vi "Main.vi"() -> ()   [LabVIEW 2020, in "ChromTech Next Gen Pump.lvlib"]
uses:
  ChromTech Next Gen Pump.lvlib
  process loops/Instrument Manager/Instrument State.ctl
  process loops/UI Manager/Data Display Loop Data.ctl
  process loops/Logging/Logging Configuration.ctl
  process loops/UI Manager/UI Data.ctl
  process loops/UI Manager/UI Display State.ctl
  Typedefs/System Control Data.ctl
  <vilib>/Utility/error.llb/Error Cluster From Error Code.vi
  <vilib>/ErrorRing/Error Ring.xnode
  support/Message Queue/Message Queue.lvlib
  support/User Event - Stop/User Event - Stop.lvlib
  process loops/Instrument Manager/Instrument Manager.lvlib
  process loops/Acquisition/Acquisition.lvlib
  process loops/Remote Connection Manager/Remote Connection Manager.lvlib
  process loops/Logging/Logging.lvlib
panel:
  in  "Time Interval (sec)":i32=1200
  out "Data Graph":cluster{timestamp[], dbl[]}[](graph)
  in  "Config Log Btn":bool
  in  "Sampling rate\n(sec/sample)":dbl=5.0 min=0.1 step=0.1
  in  "Log Data":bool
  in  "Stop Btn":bool=TRUE
  in  "Run Btn":bool
  out "Data Ind":dbl format="%d psi"
  in  "Flow Rate (mL/min)":dbl format="%.3f"
  out "VISA resource":refnum<visa-resource-name>
  # "Pump Control Panel"
  # "Config"
  # "Pump Control"
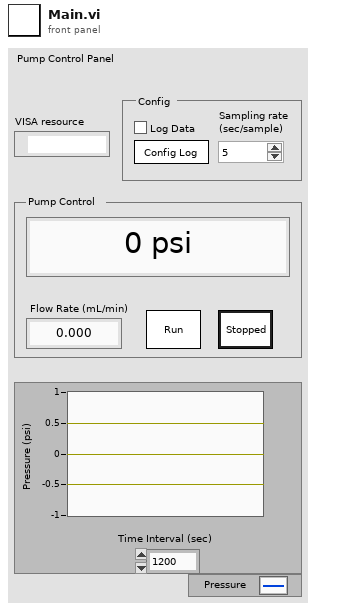
[diagram p1: front panel]
types:
  T1 = typedef "ChromTech Next Gen Pump.lvlib/Data Display Loop Data.ctl" = cluster{"Data Timestamps":timestamp[], "Data Values":dbl[], "Previous Run State":bool}
  T2 = typedef "ChromTech Next Gen Pump.lvlib/Instrument Manager.lvlib/Instrument State.ctl" = cluster{"VISA Resource":refnum<visa-resource-name>, "Flow Rate":dbl, "Running":bool, "Running Since":timestamp, "Pressure Data Point":cluster{"Time Stamp":timestamp, "Value":dbl}, "Upper Pressure Fault":bool, "Lower Pressure Fault":bool, "Motor Stall Fault":bool, "Sampling Rate (sec/sample)":dbl, "Retry Attempts":i32, "Fast Comms":bool}
  T3 = typedef "ChromTech Next Gen Pump.lvlib/Message Queue.lvlib/All Message Queues.ctl" = cluster{"System Control":refnum<queue>, "Instrument":refnum<queue>, "Remote":refnum<queue>, "UI":refnum<queue>, "Acquisition":refnum<queue>, "Logging":refnum<queue>}
  T4 = typedef "ChromTech Next Gen Pump.lvlib/UI Display State.ctl" = enum16{"Shown", "Hidden"}
  T5 = enum8{"Enabled", "Disabled", "Disabled and Grayed Out"}
  T6 = typedef "ChromTech Next Gen Pump.lvlib/UI Data.ctl" = cluster{"VISA Resource Ind":refnum<vi>, "Setpoint Ctl":refnum<vi>, "Run Btn":refnum<vi>, "Stop Btn":refnum<vi>, "Data Ind":refnum<vi>, "Log Data":refnum<vi>, "Config Log Btn":refnum<vi>, "Sampling rate\n(sec/sample)":refnum<vi>, "Data Graph":refnum<vi>}
  T7 = typedef "ChromTech Next Gen Pump.lvlib/Logging.lvlib/Logging Configuration.ctl" = cluster{"Log Directory Path":path, "Log File Path":path, "Log File Prefix":string, "Log File Extension":string, "File Delimiter":string, "Header Info":string[][], "Channels":string[], "Log Instrument Runs":bool}
  T8 = typedef "ChromTech Next Gen Pump.lvlib/System Control Data.ctl" = cluster{"Example Value <Replace Me>":dbl, "Log Runs":bool, "Clone":bool}
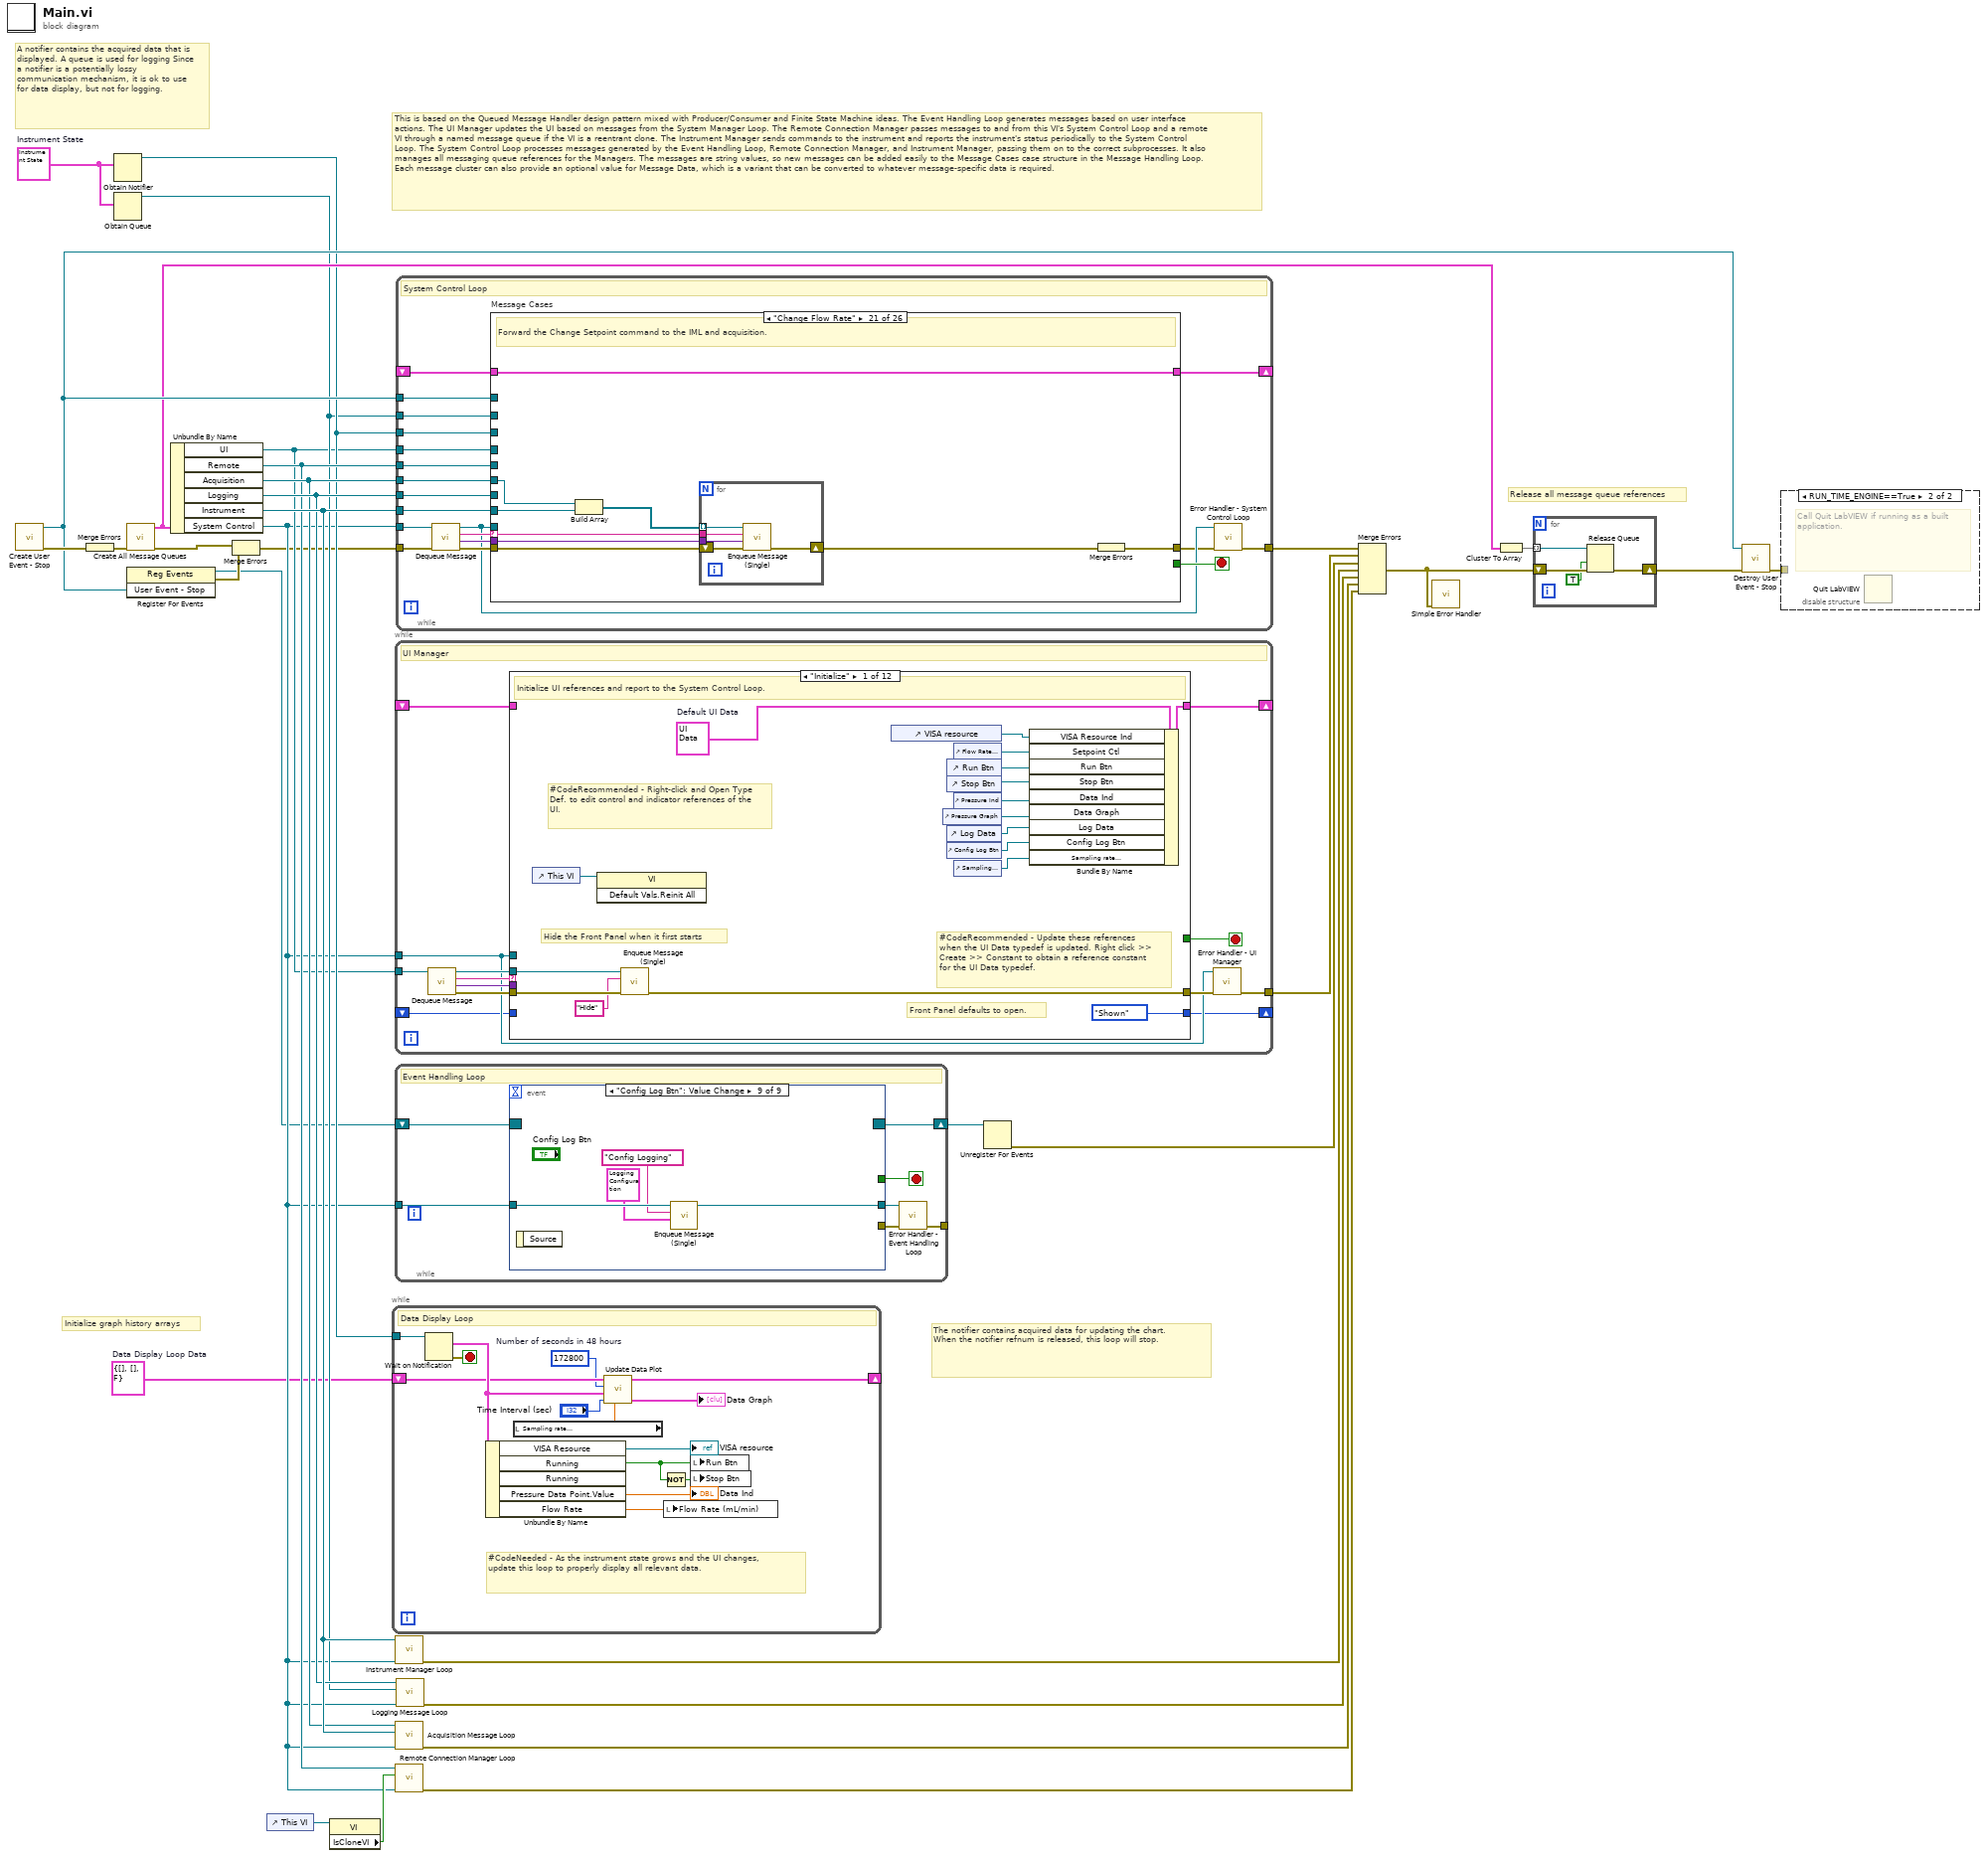
[diagram p0: block diagram]
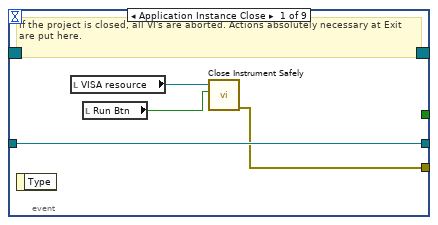
[diagram p2: hidden frame]
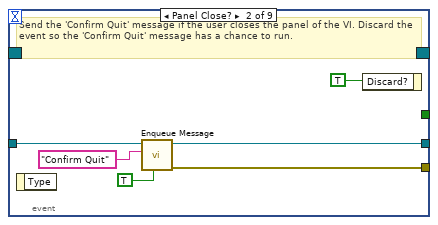
[diagram p3: hidden frame]
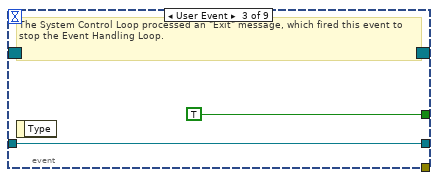
[diagram p4: hidden frame]
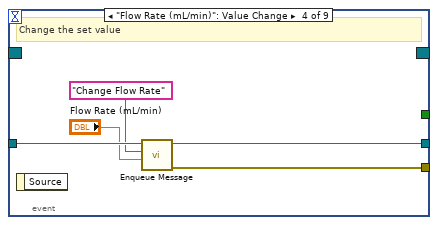
[diagram p5: hidden frame]
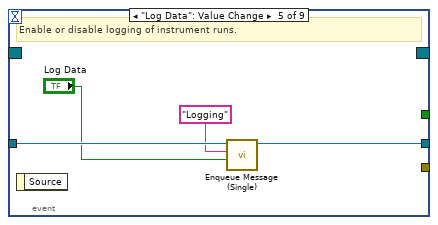
[diagram p6: hidden frame]
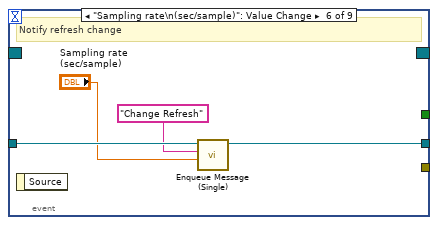
[diagram p7: hidden frame]
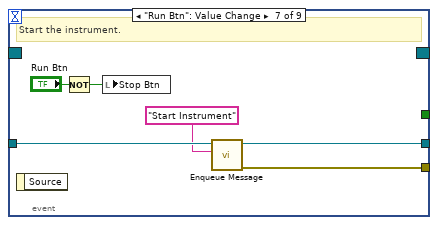
[diagram p8: hidden frame]
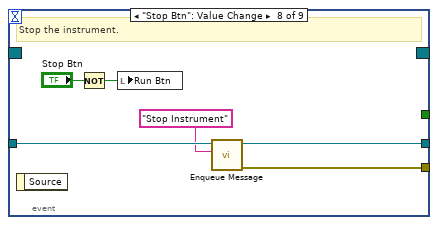
[diagram p9: hidden frame]
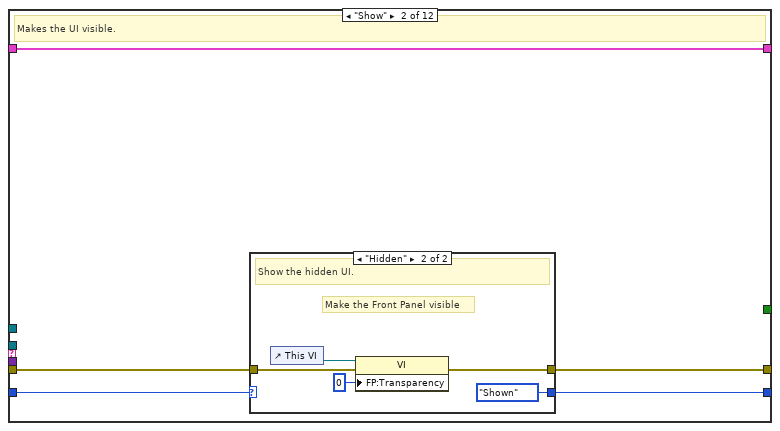
[diagram p10: hidden frame]
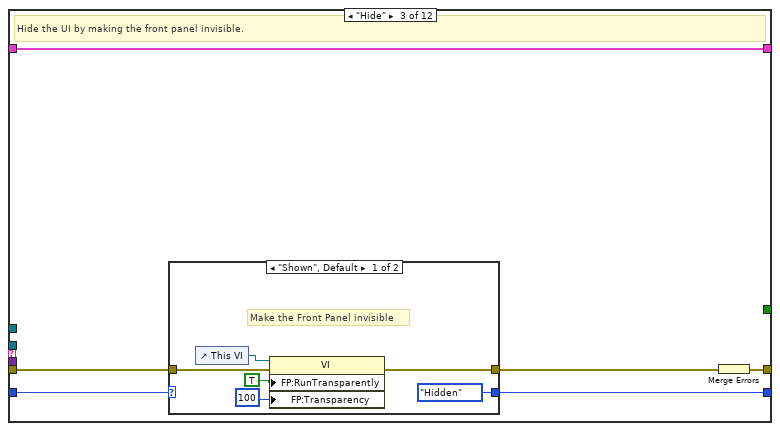
[diagram p12: hidden frame]
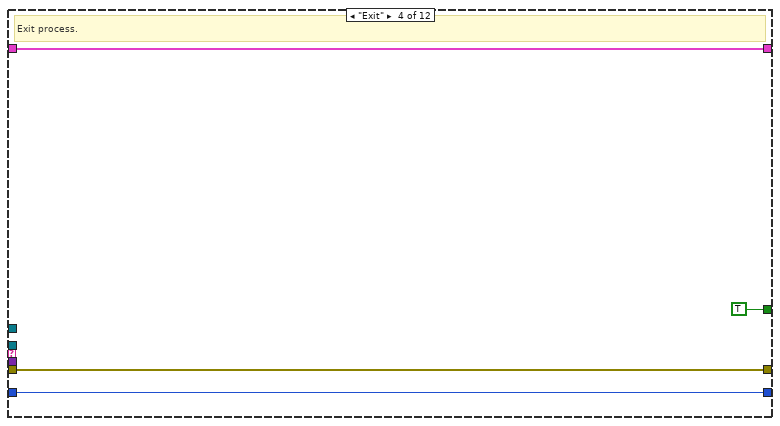
[diagram p14: hidden frame]
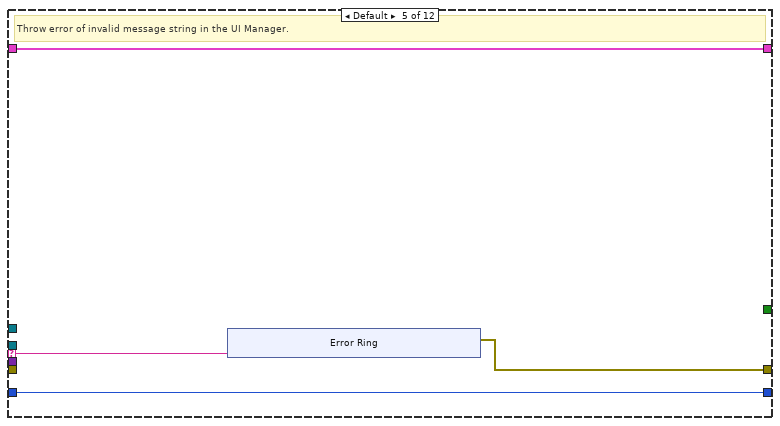
[diagram p15: hidden frame]
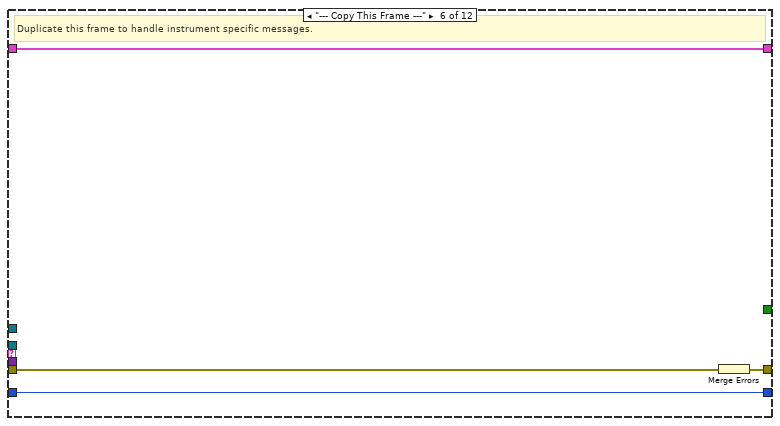
[diagram p16: hidden frame]
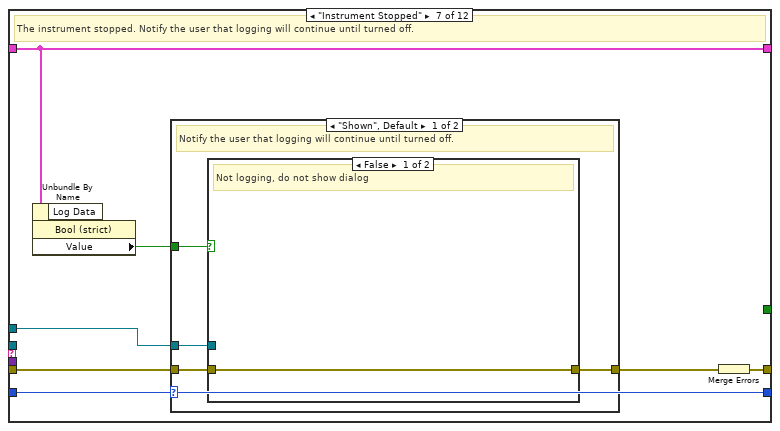
[diagram p17: hidden frame]
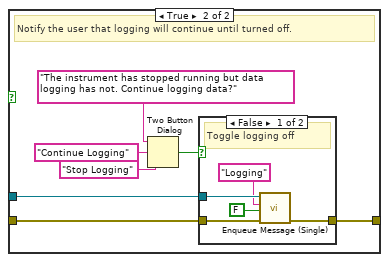
[diagram p18: hidden frame]
diagram:
  w1 = T1 {"Data Timestamps"=[], "Data Values"=[], "Previous Run State"=FALSE}  # Data Display Loop Data
  w7 = T2 {"VISA Resource"="", "Flow Rate"=0.0, "Running"=FALSE, "Running Since"=timestamp(0 s since 1904-01-01), "Pressure Data Point"={"Time Stamp"=timestamp(0 s since 1904-01-01), "Value"=0.0}, "Upper Pressure Fault"=FALSE, "Lower Pressure Fault"=FALSE, "Motor Stall Fault"=FALSE, "Sampling Rate (sec/sample)"=0.0, "Retry Attempts"=0, "Fast Comms"=FALSE}  # Instrument State
  # "Initialize graph history arrays"
  # "A notifier contains the acquired data that is displayed. A queue is used for logging Since a notifier is a potentially lossy communication mechanism, it is ok to use for data display, but not for logging."
  # "The notifier contains acquired data for updating the chart. When the notifier refnum is released, this loop will stop."
  # "Release all message queue references"
  # "This is based on the Queued Message Handler design pattern mixed with Producer/Consumer and Finite State Machine ideas. The Event Handling Loop generates messages based on user interface actions. The UI Manager updates the UI based on messages from the System Manager Loop. The Remote Connection Manager passes messages to and from this VI's System Control Loop and a remote VI through a named message queue if the VI is a reentrant clone. The Instrument Manager sends commands to the instrument and reports the instrument's status periodically to the System Control Loop. The System Control Loop processes messages generated by the Event Handling Loop, Remote Connection Manager, and Instrument Manager, passing them on to the correct subprocesses. It also manages all messaging queue references for the Managers. The messages are string values, so new messages can be added easily to the Message Cases case structure in the Message Handling Loop.  Each message cluster can also provide an optional value for Message Data, which is a variant that can be converted to whatever message-specific data is required."
  n1 = call "Create User Event - Stop.vi"() -> ("error out"=w26:errorcluster, "User Event - Stop"=w22:refnum<user-event>)  [unwired: 10 in]
  n2 = Merge Errors(w26) -> (w25:errorcluster)
  n3 = Obtain Notifier(notification data type=w7) -> (notifier out=w8:refnum<notifier>)  [unwired: 3 in, 2 out]
  n4 = Obtain Queue(element data type=w7) -> (queue out=w6:refnum<queue>)  [unwired: 4 in, 2 out]
  n5 = call "Create All Message Queues.vi"("error in (no error)"=w25) -> ("error out"=w28:errorcluster, "Message Queues out"=w11:T3)  [unwired: 9 in]
  n6 = register-events(w22) -> (reference out=w2:refnum<event-registration>, error out=w13:errorcluster)  [unwired: 2 in]
  n7 = Unbundle By Name(w11) -> ("UI"=w5:refnum<queue>, "Remote"=w29:refnum<queue>, "Acquisition"=w30:refnum<queue>, "Logging"=w31:refnum<queue>, "Instrument"=w32:refnum<queue>, "System Control"=w4:refnum<queue>)
  n8 = Merge Errors(w28, w13) -> (w3:errorcluster)
  n9 = control-ref of="This VI"() -> (w21:refnum<vi>)
  n10 = property class="VI"(reference=w21) -> ("IsCloneVI"=w20:bool)  [unwired: 1 in, 2 out]
  n11 = while "Data Display Loop" {
    tunnel: w8 -> [w46]
    shift-right: [w36] -> _
    shift-left: w1 -> [w37]
    stop <- w45 stop-if-true
    w33 = 172800  # Number of seconds in 48 hours
    # "#CodeNeeded - As the instrument state grows and the UI changes, update this loop to properly display all relevant data."
    # "Data Display Loop"
    n12 = Wait on Notification(notifier=w46) -> (notification=w38:T2, error out=w45:errorcluster)  [unwired: 3 in, 2 out]
    n13 = Unbundle By Name(w38) -> ("VISA Resource"=→"VISA resource":refnum<visa-resource-name>, "Running"=w43:bool, "Pressure Data Point.Value"=→"Data Ind":dbl, "Flow Rate"=w40:dbl)  [unwired: 1 out]
    n14 = local read "Sampling rate\n(sec/sample)"() -> (w34:dbl)
    n15 = call "Update Data Plot.vi"("Sample Rate (sec/sample)"=w34, "Time interval (s)"="Time Interval (sec)", "Instrument State"=w38, "History length (-1; unlimited)"=w33, "Graph History Arrays in"=w37) -> ("Updated Plot History"=→"Data Graph":cluster{timestamp[], dbl[]}[], "Graph History Arrays out"=w36:T1)  [unwired: 5 in]
    n16 = Not(x=w43) -> (.not. x?=w42:bool)
    n17 = local write "Flow Rate (mL/min)"(w40) -> ()
    n18 = local write "Run Btn"(w43) -> ()
    n19 = local write "Stop Btn"(w42) -> ()
  }
  n20 = while {
    tunnel: w5 -> [w59]
    tunnel: w4 -> [w50]
    tunnel: [w51] -> w19
    shift-right: [w54] -> _
    shift-left: _ -> [w53]
    shift-right: [w48] -> _
    shift-left: _ -> [w47]
    stop <- w49 stop-if-true
    # "UI Manager"
    n21 = call "Dequeue Message.vi"("Message Queue"=w59) -> ("error out"=w57:errorcluster, "Message Data"=w55:variant, "Message"=w56:string, "dup Message Queue"=w58:refnum<queue>)  [unwired: 7 in]
    n22 = case shown="\"Initialize\"" w56 {
      selector: w56 -> [_ _ _ _ w110 _ _ _ _ _ _ _]
      tunnel: w58 -> [w67 _ _ _ _ _ _ _ _ _ _ _]
      tunnel: w57 -> [w73 w80 w92 w106 _ w119 w127 w155 w163 w171 w186 w197]
      tunnel: w55 -> [_ _ _ _ _ _ _ _ _ w170 w184 w196]
      tunnel: w50 -> [_ _ _ _ _ _ w125 _ _ _ _ _]
      tunnel: [w68 w79 w93 w106 w109 w120 w129 w156 w164 w172 w187 w198] -> w52
      tunnel: [w75 w81 w94 w105 w108 w121 w124 w151 w157 w166 w179 w192] -> w54
      tunnel: w53 -> [_ w81 w94 w105 w108 w121 w124 w151 w157 w166 w179 w192]
      tunnel: [_ _ _ TRUE _ _ _ _ _ _ _ _] -> w49
      tunnel: w47 -> [_ w78 w90 w103 w107 w118 w128 w154 w162 w168 w180 w193]
      tunnel: [UI_Display_State."Shown" ("UI Display State") w77 w89 w103 w107 w118 w128 w154 w162 w168 w180 w193] -> w48
      frame "Initialize" {
        w76 = T6 {"VISA Resource Ind"=refnum, "Setpoint Ctl"=refnum, "Run Btn"=refnum, "Stop Btn"=refnum, "Data Ind"=refnum, "Log Data"=refnum, "Config Log Btn"=refnum, "Sampling rate\n(sec/sample)"=refnum, "Data Graph"=refnum}  # Default UI Data
        # "Front Panel defaults to open."
        # "Hide the Front Panel when it first starts"
        # "#CodeRecommended - Update these references when the UI Data typedef is updated. Right click >> Create >> Constant to obtain a reference constant for the UI Data typedef."
        # "#CodeRecommended - Right-click and Open Type Def. to edit control and indicator references of the UI."
        # "Initialize UI references and report to the System Control Loop."
        n23 = control-ref of="This VI"() -> (w60:refnum<vi>)
        n24 = invoke class="VI" method="Default Vals.Reinit All"(reference=w60) -> ()  [unwired: 2 in, 3 out]
        n25 = call "Enqueue Message (Single).vi"("error in (no error)"=w73, "Message"="Hide", "Message Queue"=w67) -> ("error out"=w68:errorcluster)  [unwired: 7 in, 1 out]
        n26 = control-ref of="VISA resource"() -> (w72:refnum<vi>)
        n27 = control-ref of="Pressure Graph"() -> (w64:refnum<vi>)
        n28 = control-ref of="Run Btn"() -> (w70:refnum<vi>)
        n29 = control-ref of="Stop Btn"() -> (w71:refnum<vi>)
        n30 = control-ref of="Log Data"() -> (w63:refnum<vi>)
        n31 = control-ref of="Config Log Btn"() -> (w62:refnum<vi>)
        n32 = control-ref of="Flow Rate (mL/min)"() -> (w74:refnum<vi>)
        n33 = control-ref of="Pressure Ind"() -> (w69:refnum<vi>)
        n34 = control-ref of="Sampling rate (sec/sample)"() -> (w61:refnum<vi>)
        n35 = Bundle By Name(cluster=w76, "VISA Resource Ind"=w72, "Setpoint Ctl"=w74, "Run Btn"=w70, "Stop Btn"=w71, "Data Ind"=w69, "Data Graph"=w64, "Log Data"=w63, "Config Log Btn"=w62, "Sampling rate\n(sec/sample)"=w61) -> (w75:T6)
      }
      frame "Show" {
        # "Makes the UI visible."
        n36 = case shown="\"Hidden\"" w78 {
          selector: w78 -> [w83 _]
          tunnel: w80 -> [w82 w88]
          tunnel: [w82 w86] -> w79
          tunnel: [w83 UI_Display_State."Shown" ("UI Display State")] -> w77
          frame "Shown", Default {
            # "Do nothing if UI is already shown."
          }
          frame "Hidden" {
            # "Make the Front Panel visible"
            # "Show the hidden UI."
            n37 = control-ref of="This VI"() -> (w87:refnum<vi>)
            n38 = property class="VI"(reference=w87, error in=w88, "FP:Transparency"=u8 0 ("Front Panel Window:Transparency")) -> (error out=w86:errorcluster)  [unwired: 1 out]
          }
        }
      }
      frame "Hide" {
        # "Hide the UI by making the front panel invisible."
        n39 = case shown="\"Shown\", Default" w90 {
          selector: w90 -> [_ w102]
          tunnel: w92 -> [w97 w101]
          tunnel: [w96 w101] -> w91
          tunnel: [UI_Display_State."Hidden" ("UI Display State") w102] -> w89
          frame "Shown", Default {
            # "Make the Front Panel invisible"
            n40 = control-ref of="This VI"() -> (w100:refnum<vi>)
            n41 = property class="VI"(reference=w100, error in=w97, "FP:RunTransparently"=TRUE ("Front Panel Window:Run VI Transparently"), "FP:Transparency"=u8 100 ("Front Panel Window:Transparency")) -> (error out=w96:errorcluster)  [unwired: 1 out]
          }
          frame "Hidden" {
          }
        }
        n42 = Merge Errors(w91) -> (w93:errorcluster)
      }
      frame "Exit" {
        # "Exit process."
      }
      frame Default {
        # "Throw error of invalid message string in the UI Manager."
        n43 = xnode "Error Ring"("parameter 0"=w110) -> ("error out"=w109:errorcluster)
      }
      frame "--- Copy This Frame ---" {
        # "Duplicate this frame to handle instrument specific messages."
        n44 = Merge Errors(w119) -> (w120:errorcluster)
      }
      frame "Instrument Stopped" {
        # "The instrument stopped. Notify the user that logging will continue until turned off."
        n45 = Unbundle By Name(w124) -> ("Log Data"=w123:refnum<vi>)
        n46 = property class="Bool (strict)"(reference=w123) -> ("Value"=w122:bool)  [unwired: 1 in, 2 out]
        n47 = case shown="\"Shown\", Default" w128 {
          tunnel: w127 -> [w133 w148]
          tunnel: [w132 w148] -> w126
          tunnel: w125 -> [w131 _]
          tunnel: w122 -> [w130 _]
          frame "Shown", Default {
            # "Notify the user that logging will continue until turned off."
            n48 = case shown="False" w130 {
              tunnel: w133 -> [w134 w137]
              tunnel: [w134 w136] -> w132
              tunnel: w131 -> [_ w135]
              frame False {
                # "Not logging, do not show dialog"
              }
              frame True {
                # "Notify the user that logging will continue until turned off."
                n49 = Two Button Dialog(message="The instrument has stopped running but data logging has not. Continue logging data?", 1:"Stop Logging" ("F button name (\"Cancel\")"), 2:"Continue Logging" ("T button name (\"OK\")")) -> (T button?=w138:bool)
                n50 = case shown="False" w138 {
                  tunnel: w137 -> [w146 w147]
                  tunnel: [w145 w147] -> w136
                  tunnel: w135 -> [w144 _]
                  frame False {
                    # "Toggle logging off"
                    n51 = call "Enqueue Message (Single).vi"("error in (no error)"=w146, "Message Data"=FALSE, "Message"="Logging", "Message Queue"=w144) -> ("error out"=w145:errorcluster)  [unwired: 6 in, 1 out]
                  }
                  frame True {
                    # "Continues logging. Do nothing more"
                  }
                }
              }
            }
          }
          frame "Hidden" {
            # "Hidden, do not show dialog"
          }
        }
        n52 = Merge Errors(w126) -> (w129:errorcluster)
      }
      frame "Logging Started" {
        # "Indicate that logging started."
        n53 = Unbundle By Name(w151) -> ("Log Data"=w153:refnum<vi>)
        n54 = property class="Bool (strict)"(reference=w153, "Value"=TRUE ("Log Data")) -> ()  [unwired: 1 in, 2 out]
        n55 = Unbundle By Name(w151) -> ("Config Log Btn"=w150:refnum<vi>)
        n56 = property class="Bool"(reference=w150, "DisabledEnum"=T5."Disabled and Grayed Out" ("Disabled")) -> ()  [unwired: 1 in, 2 out]
        n57 = Merge Errors(w155) -> (w156:errorcluster)
      }
      frame "Logging Stopped" {
        # "Indicate that logging stopped."
        n58 = Unbundle By Name(w157) -> ("Log Data"=w161:refnum<vi>)
        n59 = property class="Bool (strict)"(reference=w161, "Value"=FALSE ("Log Data")) -> ()  [unwired: 1 in, 2 out]
        n60 = Unbundle By Name(w157) -> ("Config Log Btn"=w159:refnum<vi>)
        n61 = property class="Bool"(reference=w159, "DisabledEnum"=T5."Enabled" ("Disabled")) -> ()  [unwired: 1 in, 2 out]
        n62 = Merge Errors(w163) -> (w164:errorcluster)
      }
      frame "Change Refresh" {
        # "Update sample rate multiplier in the UI data chart and config indicator."
        n63 = Unbundle By Name(w166) -> ("Sampling rate\n(sec/sample)"=w167:refnum<vi>)
        n64 = Variant To Data(type=0.0, Variant=w170) -> (data=w165:dbl)  [unwired: 1 in, 1 out]
        n65 = property class="DigNum (strict)"(reference=w167, "Value"=w165) -> ()  [unwired: 1 in, 2 out]
        n66 = Merge Errors(w171) -> (w172:errorcluster)
      }
      frame "Update Pressure Units" {
        # "Change the units of the display."
        n67 = Variant To Data(type="", Variant=w184) -> (data=w174:string)  [unwired: 1 in, 1 out]
        n68 = call <vilib>:"Space Constant.vi"() -> ("String"=w183:string)
        n69 = Concatenate Strings("%d" ("string"), w183, w174) -> (w181:string)
        n70 = Unbundle By Name(w179) -> ("Data Ind"=w178:refnum<vi>, "Data Graph"=w173:refnum<vi>)
        n71 = Concatenate Strings("Pressure (" ("concatenated string"), w174, ")" ("string")) -> (w177:string)
        n72 = property on="Property Node" class="DigNum (strict)"(reference=w178, "FormatString"=w181) -> ()  [unwired: 1 in, 2 out]
        n73 = property class="XYGraph (strict)"(reference=w173, "YScale.NameLbl.Text"=w177) -> ()  [unwired: 1 in, 2 out]
        n74 = Merge Errors(w186) -> (w187:errorcluster)
      }
      frame "Update Flow Rate Units" {
        # "Change the units of the setpoint display."
        n75 = Variant To Data(type="", Variant=w196) -> (data=w190:string)  [unwired: 1 in, 1 out]
        n76 = Concatenate Strings("Flow Rate (" ("string"), w190, ")" ("string")) -> (w194:string)
        n77 = Unbundle By Name(w192) -> ("Setpoint Ctl"=w191:refnum<vi>)
        n78 = property on="Property Node" class="DigNum (strict)"(reference=w191, "FormatString"=w194) -> ()  [unwired: 1 in, 2 out]
        n79 = Merge Errors(w197) -> (w198:errorcluster)
      }
    }
    n80 = call "Error Handler - UI Manager.vi"("error in (no error)"=w52, "Message Queue"=w50) -> ("dup error in"=w51:errorcluster)  [unwired: 8 in, 1 out]
  }
  n81 = while {
    tunnel: w4 -> [w205]
    shift-right: [w203] -> w23
    shift-left: w2 -> [w204]
    tunnel: [w199] -> _
    stop <- w201 stop-if-true
    # "Event Handling Loop"
    n82 = event shown="[8] \"Config Log Btn\": Value Change" {
      selector: w204 -> [_ _ _ _ _ _ _ _ _]
      dyn-events: [_ _ _ _ _ _ _ _ _] -> w203
      timeout: _ -> [_ _ _ _ _ _ _ _ _]
      tunnel: [_ _ TRUE ("Discard?") _ _ _ _ _ _] -> w201
      tunnel: w205 -> [w209 w214 w217 w222 w226 w230 w236 w242 w246]
      tunnel: [w208 w213 _ w219 _ _ w234 w240 _] -> w202
      tunnel: [w209 w212 w217 w221 w225 w229 w235 w241 w245] -> w200
      event Application Instance Close {
        # "If the project is closed, all VI's are aborted. Actions absolutely necessary at Exit are put here."
        n83 = event-data() -> ()  [unwired: 1 in, 1 out]
        n84 = local read "VISA resource"() -> (w207:refnum<visa-resource-name>)
        n85 = local read "Run Btn"() -> (w206:bool)
        n86 = call "Close Instrument Safely.vi"("Running (F)"=w206, "VISA Refnum in"=w207) -> ("error out"=w208:errorcluster)  [unwired: 9 in]
      }
      event Panel Close? {
        # "Send the 'Confirm Quit' message if the user closes the panel of the VI. Discard the event so the 'Confirm Quit' message has a chance to run."
        n87 = event-data() -> ()  [unwired: 1 in, 1 out]
        n88 = call-poly "Enqueue Message.vi"("Priority Message? (F)"=TRUE, "Message"="Confirm Quit", "Message Queue"=w214) -> ("error out"=w213:errorcluster, "dup Message Queue"=w212:refnum<queue>)  [unwired: 7 in]
        n89 = event-data("Discard?"=TRUE) -> ()  [unwired: 1 in, 1 out]
      }
      event User Event {
        # "The System Control Loop processed an \"Exit\" message, which fired this event to stop the Event Handling Loop."
        n90 = event-data() -> ()  [unwired: 1 in, 1 out]
      }
      event "Flow Rate (mL/min)": Value Change {
        # "Change the set value"
        n91 = event-data() -> ()  [unwired: 1 in, 1 out]
        n92 = call-poly "Enqueue Message.vi"("Message Data"="Flow Rate (mL/min)", "Message"="Change Flow Rate", "Message Queue"=w222) -> ("error out"=w219:errorcluster, "dup Message Queue"=w221:refnum<queue>)  [unwired: 7 in]
      }
      event "Log Data": Value Change {
        # "Enable or disable logging of instrument runs."
        n93 = event-data() -> ()  [unwired: 1 in, 1 out]
        n94 = call "Enqueue Message (Single).vi"("Message Data"="Log Data", "Message"="Logging", "Message Queue"=w226) -> ("dup Message Queue"=w225:refnum<queue>)  [unwired: 7 in, 1 out]
      }
      event "Sampling rate\n(sec/sample)": Value Change {
        # "Notify refresh change"
        n95 = event-data() -> ()  [unwired: 1 in, 1 out]
        n96 = call "Enqueue Message (Single).vi"("Message Data"="Sampling rate\n(sec/sample)", "Message"="Change Refresh", "Message Queue"=w230) -> ("dup Message Queue"=w229:refnum<queue>)  [unwired: 7 in, 1 out]
      }
      event "Run Btn": Value Change {
        # "Start the instrument."
        n97 = event-data() -> ()  [unwired: 1 in, 1 out]
        n98 = Not(x="Run Btn") -> (.not. x?=w231:bool)
        n99 = local write "Stop Btn"(w231) -> ()
        n100 = call-poly "Enqueue Message.vi"("Message"="Start Instrument", "Message Queue"=w236) -> ("error out"=w234:errorcluster, "dup Message Queue"=w235:refnum<queue>)  [unwired: 8 in]
      }
      event "Stop Btn": Value Change {
        # "Stop the instrument."
        n101 = event-data() -> ()  [unwired: 1 in, 1 out]
        n102 = Not(x="Stop Btn") -> (.not. x?=w237:bool)
        n103 = local write "Run Btn"(w237) -> ()
        n104 = call-poly "Enqueue Message.vi"("Message"="Stop Instrument", "Message Queue"=w242) -> ("error out"=w240:errorcluster, "dup Message Queue"=w241:refnum<queue>)  [unwired: 8 in]
      }
      event "Config Log Btn": Value Change {
        n105 = event-data() -> ()  [unwired: 1 in, 1 out]
        n106 = call "Enqueue Message (Single).vi"("Message Data"=T7 {"Log Directory Path"=path "", "Log File Path"=path "", "Log File Prefix"="Experiment", "Log File Extension"="csv", "File Delimiter"=",", "Header Info"=[], "Channels"=[], "Log Instrument Runs"=FALSE} ("Logging Configuration"), "Message"="Config Logging", "Message Queue"=w246) -> ("dup Message Queue"=w245:refnum<queue>)  [unwired: 7 in, 1 out]
      }
    }
    n107 = call "Error Handler - Event Handling Loop.vi"("error in (no error)"=w202, "Message Queue"=w200) -> ("dup error in"=w199:errorcluster)  [unwired: 8 in, 1 out]
  }
  n108 = call "Instrument Manager Loop.vi"("System Control"=w4, "Instrument Manager"=w32) -> ("error out"=w17:errorcluster)  [unwired: 9 in]
  n109 = call "Acquisition Message Loop.vi"("System Control"=w4, "Instrument Manager"=w32, "Acquisition"=w30) -> ("error out"=w15:errorcluster)  [unwired: 8 in]
  n110 = call "Remote Connection Manager Loop.vi"("System Control"=w4, "IsCloneVI (false)"=w20, "Remote"=w29) -> ("error out"=w14:errorcluster)  [unwired: 8 in]
  n111 = while {
    tunnel: w4 -> [w257]
    shift-right: [w264] -> _
    shift-left: _ -> [w265]
    tunnel: w22 -> [w262]
    tunnel: w3 -> [w261]
    tunnel: [w255] -> w27
    tunnel: w32 -> [w253]
    tunnel: w29 -> [w252]
    tunnel: w5 -> [w251]
    tunnel: w30 -> [w250]
    tunnel: w31 -> [w249]
    tunnel: w8 -> [w248]
    tunnel: w6 -> [w247]
    stop <- w263 stop-if-true
    # "System Control Loop"
    n112 = call "Dequeue Message.vi"("error in (no error)"=w261, "Message Queue"=w257) -> ("error out"=w260:errorcluster, "Message Data"=w258:variant, "Message"=w259:string, "dup Message Queue"=w256:refnum<queue>)  [unwired: 6 in]
    n113 = case "Message Cases" shown="\"Change Flow Rate\"" w259 {
      selector: w259 -> [_ _ _ w307 w320 w331 w351 w366 w379 w393 w399 _ w445 w452 w459 w466 w473 w483 w497 w512 w526 w537 w544 w554 w569 w591]
      tunnel: w256 -> [_ _ w287 _ _ _ _ _ _ _ _ _ _ _ _ _ _ _ _ _ _ _ _ _ _ _]
      tunnel: w260 -> [w269 w284 w291 _ _ w334 w354 w369 w382 w397 w415 w428 w449 w456 w463 w470 w477 w486 w500 w516 w530 w540 w547 _ _ _]
      tunnel: [w268 w278 w289 w310 w321 w340 w355 w370 w384 w398 w406 w433 w450 w457 w464 w471 w478 w487 w501 w514 w528 w541 w548 w553 w568 w590] -> w254
      tunnel: w265 -> [_ w283 w290 w306 w322 w341 w356 w371 w385 w396 w405 w434 w451 w458 w465 w472 w479 w488 w502 w515 w529 w542 w549 w552 w565 w588]
      tunnel: [w270 w283 w290 w306 w322 w341 w356 w371 w385 w396 w405 w432 w451 w458 w465 w472 w479 w488 w502 w515 w529 w542 w549 w552 w565 w588] -> w264
      tunnel: [_ _ _ TRUE _ _ _ _ _ _ _ _ _ _ _ _ _ _ _ _ _ _ _ _ _ _] -> w263
      tunnel: w258 -> [_ w282 _ w311 _ w330 w350 w365 w378 w392 w400 w430 w446 w453 w460 w467 w474 w484 w498 w511 w525 w538 w545 w555 w570 w586]
      tunnel: w262 -> [_ _ _ w308 _ _ _ _ _ _ _ _ _ _ _ _ _ _ _ _ _ _ _ _ _ _]
      tunnel: w253 -> [w267 _ _ w303 _ w335 _ _ _ w394 _ _ _ _ _ _ _ _ _ _ w524 w536 w543 _ _ _]
      tunnel: w252 -> [_ _ _ w302 _ w338 _ _ w383 _ w410 _ _ _ _ _ _ w482 w496 _ _ _ _ w556 w566 w589]
      tunnel: w251 -> [_ _ _ w301 _ w337 w348 w363 _ _ w409 _ _ _ _ _ _ w481 w495 w509 _ _ _ _ w564 _]
      tunnel: w250 -> [_ _ _ w305 _ w339 _ _ _ _ w412 _ _ _ _ _ _ _ _ w510 w523 _ _ w551 _ _]
      tunnel: w249 -> [_ _ _ w304 _ w336 w349 w364 _ _ w402 w426 w447 w454 w461 w468 w475 _ _ _ _ _ _ w550 _ _]
      tunnel: w248 -> [_ _ _ w298 _ _ _ _ _ _ _ _ _ _ _ _ _ _ _ _ _ _ _ _ _ w587]
      tunnel: w247 -> [_ _ _ w296 _ _ _ _ _ _ _ _ _ _ _ _ _ _ _ _ _ _ _ _ _ w583]
      frame "Initialize" {
        w271 = T8 {"Example Value <Replace Me>"=0.0, "Log Runs"=FALSE, "Clone"=FALSE}  # Default Data
        # "Initialize the system control loop and system."
        n114 = control-ref of="This VI"() -> ()  [unwired: 1 out]
        n115 = property on="Property Node" class="VI"() -> ("IsCloneVI"=w266:bool)  [unwired: 2 in, 2 out]
        n116 = Bundle By Name(cluster=w271, "Clone"=w266) -> (w270:T8)
        n117 = case shown="False" w266 {
          tunnel: w269 -> [w274 w277]
          tunnel: [w273 w277] -> w268
          tunnel: w267 -> [w272 _]
          frame False {
            # "Initiate the VISA Resource selection window if this is not a"
            n118 = call "Enqueue Message (Single).vi"("error in (no error)"=w274, "Message Data"=refnum<visa-resource-name> refnum ("VISA resource out"), "Message"="Set VISA Resource", "Message Queue"=w272) -> ("error out"=w273:errorcluster)  [unwired: 6 in, 1 out]
          }
          frame True {
            # "Reentrant clone. It is the responsibility of the RCM to send the Set VISA Resource command."
          }
        }
      }
      frame "Error" {
        # "#CodeRecommended - If you ever change the name of this \"Error\" message, you'll need to update the name in the Check Loop Error.vi as well."
        # "#CodeRecommended - Consider creating a system for logging errors in some way. These errors are for notification purposes only. Handling of specific errors should be performed in the message frames that generated the error."
        # "Error - Display an error dialog. This message is sent by the \"Error Handler\" VIs at the end of other loops in this application."
        n119 = Variant To Data(error in=w284, type=errorcluster {"status"=FALSE, "code"=0, "source"=""} ("error constant"), Variant=w282) -> (data=w280:errorcluster, error out=w279:errorcluster)
        n120 = call <vilib>:"Simple Error Handler.vi"("error in (no error)"=w280) -> ()  [unwired: 4 in, 5 out]
        n121 = Merge Errors(w279) -> (w278:errorcluster)
      }
      frame "Confirm Quit" {
        # "#CodeNeeded - If you want to provide an \"Are you sure\" dialog (or some other notification) before the application exits, place that code here. This message is typically sent from a Panel Close? event."
        # "Confirm Quit - Message that can confirm whether or not the user wants to exit the application."
        n122 = call-poly "Enqueue Message.vi"("Priority Message? (F)"=TRUE, "error in (no error)"=w291, "Message"="Exit", "Message Queue"=w287) -> ("error out"=w288:errorcluster)  [unwired: 6 in, 1 out]
        n123 = Merge Errors(w288) -> (w289:errorcluster)
      }
      frame "Exit" {
        # "Order other processes to exit"
        # "Begin the application closing procedure by sending \"Exit\" commands to all running processes."
        n124 = Variant To Data(type=errorcluster {"status"=FALSE, "code"=0, "source"=""} ("error constant"), Variant=w311) -> (data=w312:errorcluster)  [unwired: 1 in, 1 out]
        n125 = Build Array(w301, w302, w305, w304, w303) -> (w300:refnum<queue>[])
        n126 = call <vilib>:"Clear Errors.vi"("error in (no error)"=w312, "specific error code to clear (0: all)"=5000) -> ("error out"=w293:errorcluster)  [unwired: 4 in, 1 out]
        n127 = call <vilib>:"Simple Error Handler.vi"("error in (no error)"=w293) -> ()  [unwired: 4 in, 5 out]
        n128 = for {
          tunnel: w307 -> [w318]
          tunnel: w300 -> [w317] mode=indexing
          shift-right: [w316] -> w309
          shift-left: _ -> [w315]
          n129 = call "Enqueue Message (Single).vi"("Priority Message? (F)"=TRUE, "Message"=w318, "Message Queue"=w317) -> ("error out"=w319:errorcluster)  [unwired: 7 in, 1 out]
          n130 = Merge Errors(w319, w315) -> (w316:errorcluster)
        }
        n131 = Release Notifier(notifier=w298) -> (error out=w297:errorcluster)  [unwired: 2 in, 2 out]
        n132 = Release Queue(queue=w296) -> (error out=w294:errorcluster)  [unwired: 2 in, 2 out]
        n133 = call "Fire User Event - Stop.vi"("User Event - Stop"=w308) -> ("error out"=w295:errorcluster)  [unwired: 10 in]
        n134 = Merge Errors(w295, w294, w297, w309) -> (w310:errorcluster)
      }
      frame Default {
        # "'Default' case only runs if there is a message that isn't defined in any of the other cases.  Output a programming error."
        n135 = xnode "Error Ring"("parameter 0"=w320) -> ("error out"=w321:errorcluster)
      }
      frame "---Copy This Frame---" {
        # "Sends the message to each process in the array."
        # "#CodeRecommended - Change connections to build an array of the processes that will receive this message"
        # "Duplicate this frame when creating new messages.  Change this comment in the duplicated frame to describe this message."
        n136 = Build Array(w337, w338, w339, w336, w335) -> (w332:refnum<queue>[])
        n137 = for {
          tunnel: w332 -> [w345] mode=indexing
          tunnel: w331 -> [w347]
          tunnel: w330 -> [w346]
          shift-right: [w344] -> w333
          shift-left: w334 -> [w342]
          n138 = call "Enqueue Message (Single).vi"("Message Data"=w346, "Message"=w347, "Message Queue"=w345) -> ("error out"=w343:errorcluster)  [unwired: 7 in, 1 out]
          n139 = Merge Errors(w343, w342) -> (w344:errorcluster)
        }
        n140 = Merge Errors(w333) -> (w340:errorcluster)
      }
      frame "Update Pressure Units" {
        # "Sends the message to each process in the array."
        # "Change the pressure units."
        n141 = Build Array(w348, w349) -> (w352:refnum<queue>[])
        n142 = for {
          tunnel: w352 -> [w360] mode=indexing
          tunnel: w351 -> [w362]
          tunnel: w350 -> [w361]
          shift-right: [w359] -> w353
          shift-left: w354 -> [w357]
          n143 = call "Enqueue Message (Single).vi"("Message Data"=w361, "Message"=w362, "Message Queue"=w360) -> ("error out"=w358:errorcluster)  [unwired: 7 in, 1 out]
          n144 = Merge Errors(w358, w357) -> (w359:errorcluster)
        }
        n145 = Merge Errors(w353) -> (w355:errorcluster)
      }
      frame "Update Flow Rate Units" {
        # "Sends the message to each process in the array."
        # "Change the flow rate units."
        n146 = Build Array(w363, w364) -> (w367:refnum<queue>[])
        n147 = for {
          tunnel: w367 -> [w375] mode=indexing
          tunnel: w366 -> [w377]
          tunnel: w365 -> [w376]
          shift-right: [w374] -> w368
          shift-left: w369 -> [w372]
          n148 = call "Enqueue Message (Single).vi"("Message Data"=w376, "Message"=w377, "Message Queue"=w375) -> ("error out"=w373:errorcluster)  [unwired: 7 in, 1 out]
          n149 = Merge Errors(w373, w372) -> (w374:errorcluster)
        }
        n150 = Merge Errors(w368) -> (w370:errorcluster)
      }
      frame "Set Remote Queue" {
        # "Sends the message to each process in the array."
        # "Bounce this message back to the Remote Control Manager to set the remote queue to publish messages to."
        n151 = Build Array(w383) -> (w380:refnum<queue>[])
        n152 = for {
          tunnel: w380 -> [w389] mode=indexing
          tunnel: w379 -> [w391]
          tunnel: w378 -> [w390]
          shift-right: [w388] -> w381
          shift-left: w382 -> [w386]
          n153 = call "Enqueue Message (Single).vi"("Message Data"=w390, "Message"=w391, "Message Queue"=w389) -> ("error out"=w387:errorcluster)  [unwired: 7 in, 1 out]
          n154 = Merge Errors(w387, w386) -> (w388:errorcluster)
        }
        n155 = Merge Errors(w381) -> (w384:errorcluster)
      }
      frame "Set VISA Resource" {
        # "Update the VISA Resource of the instrument."
        n156 = call "Enqueue Message (Single).vi"("error in (no error)"=w397, "Message Data"=w392, "Message"=w393, "Message Queue"=w394) -> ("error out"=w395:errorcluster)  [unwired: 6 in, 1 out]
        n157 = Merge Errors(w395) -> (w398:errorcluster)
      }
      frame "Valid VISA Resource" {
        # "When a Valid VISA Resource has been chosen, start the other processes."
        n158 = Unbundle By Name(w405) -> ("Log Runs"=w404:bool)
        n159 = call "Enqueue Message (Single).vi"("error in (no error)"=w415, "Message Data"=w400, "Message"=w399, "Message Queue"=w402) -> ("error out"=w403:errorcluster, "dup Message Queue"=w401:refnum<queue>)  [unwired: 6 in]
        n160 = case shown="True" w404 {
          tunnel: w403 -> [w416 w420]
          tunnel: w401 -> [_ w419]
          tunnel: [w416 w417] -> w413
          frame False {
          }
          frame True {
            n161 = call "Enqueue Message (Single).vi"("error in (no error)"=w420, "Message"="Start", "Message Queue"=w419) -> ("error out"=w417:errorcluster)  [unwired: 7 in, 1 out]
          }
        }
        n162 = call "Enqueue Message (Single).vi"("error in (no error)"=w413, "Message"="Start", "Message Queue"=w412) -> ("error out"=w411:errorcluster)  [unwired: 7 in, 1 out]
        n163 = Unbundle By Name(w405) -> ("Clone"=w407:bool)
        n164 = call "Enqueue Message (Single).vi"("error in (no error)"=w411, "Message Data"=w400, "Message"=w399, "Message Queue"=w410) -> ("error out"=w408:errorcluster)  [unwired: 6 in, 1 out]
        n165 = case shown="False" w407 {
          tunnel: w408 -> [w424 w425]
          tunnel: [w423 w425] -> w406
          tunnel: w409 -> [w422 _]
          frame False {
            # "Show the Front Panel automatically on startup"
            n166 = call "Enqueue Message (Single).vi"("error in (no error)"=w424, "Message"="Show", "Message Queue"=w422) -> ("error out"=w423:errorcluster)  [unwired: 7 in, 1 out]
          }
          frame True {
            # "Reentrant clone. It is the responsibility of the RCM to send \"Show\"."
          }
        }
      }
      frame "Logging" {
        # "Enable or disable logging in the System Data. Run logging is disabled by default."
        n167 = Variant To Data(type=TRUE, Variant=w430) -> (data=w429:bool)  [unwired: 1 in, 1 out]
        n168 = case shown="True" w429 {
          tunnel: w428 -> [w439 w444]
          tunnel: [w438 w443] -> w427
          tunnel: w426 -> [w437 w442]
          frame False {
            n169 = call "Enqueue Message (Single).vi"("Priority Message? (F)"=TRUE, "error in (no error)"=w439, "Message"="Stop", "Message Queue"=w437) -> ("error out"=w438:errorcluster)  [unwired: 6 in, 1 out]
          }
          frame True {
            n170 = call "Enqueue Message (Single).vi"("Priority Message? (F)"=TRUE, "error in (no error)"=w444, "Message"="Start", "Message Queue"=w442) -> ("error out"=w443:errorcluster)  [unwired: 6 in, 1 out]
          }
        }
        n171 = Bundle By Name(cluster=w434, "Log Runs"=w429) -> (w432:T8)
        n172 = Merge Errors(w427) -> (w433:errorcluster)
      }
      frame "Config Logging" {
        # "Pass on Config Logging message to Logging Loop."
        n173 = call "Enqueue Message (Single).vi"("error in (no error)"=w449, "Message Data"=w446, "Message"=w445, "Message Queue"=w447) -> ("error out"=w448:errorcluster)  [unwired: 6 in, 1 out]
        n174 = Merge Errors(w448) -> (w450:errorcluster)
      }
      frame "Set Log Directory" {
        # "Pass on log setting message to Logging Loop."
        n175 = call "Enqueue Message (Single).vi"("error in (no error)"=w456, "Message Data"=w453, "Message"=w452, "Message Queue"=w454) -> ("error out"=w455:errorcluster)  [unwired: 6 in, 1 out]
        n176 = Merge Errors(w455) -> (w457:errorcluster)
      }
      frame "Set Log File Prefix" {
        # "Pass on log setting message to Logging Loop."
        n177 = call "Enqueue Message (Single).vi"("error in (no error)"=w463, "Message Data"=w460, "Message"=w459, "Message Queue"=w461) -> ("error out"=w462:errorcluster)  [unwired: 6 in, 1 out]
        n178 = Merge Errors(w462) -> (w464:errorcluster)
      }
      frame "Set Log File Delimiter" {
        # "Pass on log setting message to Logging Loop."
        n179 = call "Enqueue Message (Single).vi"("error in (no error)"=w470, "Message Data"=w467, "Message"=w466, "Message Queue"=w468) -> ("error out"=w469:errorcluster)  [unwired: 6 in, 1 out]
        n180 = Merge Errors(w469) -> (w471:errorcluster)
      }
      frame "Set Log on Run" {
        # "Pass on log setting message to Logging Loop."
        n181 = call "Enqueue Message (Single).vi"("error in (no error)"=w477, "Message Data"=w474, "Message"=w473, "Message Queue"=w475) -> ("error out"=w476:errorcluster)  [unwired: 6 in, 1 out]
        n182 = Merge Errors(w476) -> (w478:errorcluster)
      }
      frame "Logging Started" {
        # "Pass on Logging Started message to RCM and UI."
        n183 = Build Array(w481, w482) -> (w480:refnum<queue>[])
        n184 = for {
          tunnel: w484 -> [w491]
          tunnel: w483 -> [w490]
          shift-right: [w492] -> w485
          shift-left: w486 -> [w493]
          tunnel: w480 -> [w489] mode=indexing
          n185 = call "Enqueue Message (Single).vi"("error in (no error)"=w493, "Message Data"=w491, "Message"=w490, "Message Queue"=w489) -> ("error out"=w492:errorcluster)  [unwired: 6 in, 1 out]
        }
        n186 = Merge Errors(w485) -> (w487:errorcluster)
      }
      frame "Logging Stopped" {
        # "Pass on Logging Stopped message to RCM and UI."
        n187 = Build Array(w495, w496) -> (w494:refnum<queue>[])
        n188 = for {
          tunnel: w498 -> [w505]
          tunnel: w497 -> [w504]
          shift-right: [w506] -> w499
          shift-left: w500 -> [w507]
          tunnel: w494 -> [w503] mode=indexing
          n189 = call "Enqueue Message (Single).vi"("error in (no error)"=w507, "Message Data"=w505, "Message"=w504, "Message Queue"=w503) -> ("error out"=w506:errorcluster)  [unwired: 6 in, 1 out]
        }
        n190 = Merge Errors(w499) -> (w501:errorcluster)
      }
      frame "Change Refresh" {
        # "#CodeRecommended - If the default refresh time is changed, it must be updated in the UI and Data Acquisition Loop Data typedef."
        # "Change the sampling rate of the instrument. Default is 1 second/sample."
        n191 = Build Array(w509, w510) -> (w508:refnum<queue>[])
        n192 = for {
          tunnel: w512 -> [w519]
          tunnel: w511 -> [w518]
          tunnel: w508 -> [w517] mode=indexing
          shift-right: [w520] -> w513
          shift-left: w516 -> [w521]
          n193 = call "Enqueue Message (Single).vi"("error in (no error)"=w521, "Message Data"=w518, "Message"=w519, "Message Queue"=w517) -> ("error out"=w520:errorcluster)  [unwired: 6 in, 1 out]
        }
        n194 = Merge Errors(w513) -> (w514:errorcluster)
      }
      frame "Change Flow Rate" {
        # "Forward the Change Setpoint command to the IML and acquisition."
        n195 = Build Array(w523, w524) -> (w522:refnum<queue>[])
        n196 = for {
          tunnel: w526 -> [w533]
          tunnel: w525 -> [w532]
          shift-right: [w534] -> w527
          shift-left: w530 -> [w535]
          tunnel: w522 -> [w531] mode=indexing
          n197 = call "Enqueue Message (Single).vi"("error in (no error)"=w535, "Message Data"=w532, "Message"=w533, "Message Queue"=w531) -> ("error out"=w534:errorcluster)  [unwired: 6 in, 1 out]
        }
        n198 = Merge Errors(w527) -> (w528:errorcluster)
      }
      frame "Start Instrument" {
        # "Pass message to Instrument Manager Loop."
        n199 = call "Enqueue Message (Single).vi"("error in (no error)"=w540, "Message Data"=w538, "Message"=w537, "Message Queue"=w536) -> ("error out"=w539:errorcluster)  [unwired: 6 in, 1 out]
        n200 = Merge Errors(w539) -> (w541:errorcluster)
      }
      frame "Stop Instrument" {
        # "Pass message to Instrument Manager Loop."
        n201 = call "Enqueue Message (Single).vi"("error in (no error)"=w547, "Message Data"=w545, "Message"=w544, "Message Queue"=w543) -> ("error out"=w546:errorcluster)  [unwired: 6 in, 1 out]
        n202 = Merge Errors(w546) -> (w548:errorcluster)
      }
      frame "Instrument Started" {
        # "Build an array of all processes that will receive this message"
        # "Notify processes of update"
        # "Notify processes that the instrument is running."
        n203 = Build Array(w556, w551, w550) -> (w557:refnum<queue>[])
        n204 = for {
          tunnel: w557 -> [w561] mode=indexing
          tunnel: w554 -> [w563]
          tunnel: w555 -> [w562]
          shift-right: [w560] -> w553
          shift-left: _ -> [w558]
          n205 = call "Enqueue Message (Single).vi"("Message Data"=w562, "Message"=w563, "Message Queue"=w561) -> ("error out"=w559:errorcluster)  [unwired: 7 in, 1 out]
          n206 = Merge Errors(w559, w558) -> (w560:errorcluster)
        }
      }
      frame "Instrument Stopped" {
        # "Build an array of all processes that will receive this message"
        # "Notify processes of update"
        # "Notify processes that the instrument stopped running."
        n207 = Build Array(w564, w566) -> (w567:refnum<queue>[])
        n208 = for {
          tunnel: w567 -> [w574] mode=indexing
          tunnel: w569 -> [w576]
          tunnel: w570 -> [w575]
          shift-right: [w573] -> w568
          shift-left: _ -> [w571]
          n209 = call "Enqueue Message (Single).vi"("Message Data"=w575, "Message"=w576, "Message Queue"=w574) -> ("error out"=w572:errorcluster)  [unwired: 7 in, 1 out]
          n210 = Merge Errors(w572, w571) -> (w573:errorcluster)
        }
      }
      frame "Report" {
        # "Send instrument state notification"
        # "Notify processes that the instrument stopped running."
        n211 = Variant To Data(type=T2 {"VISA Resource"="", "Flow Rate"=0.0, "Running"=FALSE, "Running Since"=timestamp(0 s since 1904-01-01), "Pressure Data Point"={"Time Stamp"=timestamp(0 s since 1904-01-01), "Value"=0.0}, "Upper Pressure Fault"=FALSE, "Lower Pressure Fault"=FALSE, "Motor Stall Fault"=FALSE, "Sampling Rate (sec/sample)"=0.0, "Retry Attempts"=0, "Fast Comms"=FALSE} ("Instrument State"), Variant=w586) -> (data=w582:T2)  [unwired: 1 in, 1 out]
        n212 = local read "Sampling rate\n(sec/sample)"() -> (w578:dbl)
        n213 = Bundle By Name(cluster=w582, "Sampling Rate (sec/sample)"=w578) -> (w577:T2)
        n214 = Enqueue Element(queue=w583, element=w577) -> (error out=w580:errorcluster)  [unwired: 2 in, 2 out]
        n215 = Send Notification(notification=w577, notifier=w587) -> (error out=w584:errorcluster)  [unwired: 1 in, 1 out]
        n216 = Merge Errors(w580, w584) -> (w581:errorcluster)
        n217 = call "Enqueue Message (Single).vi"("Message Data"=w577, "Message"=w591, "Message Queue"=w589) -> ("error out"=w579:errorcluster)  [unwired: 7 in, 1 out]
        n218 = Merge Errors(w579, w581) -> (w590:errorcluster)
      }
    }
    n219 = call "Error Handler - System Control Loop.vi"("error in (no error)"=w254, "Message Queue"=w256) -> ("dup error in"=w255:errorcluster)  [unwired: 8 in, 1 out]
  }
  n220 = call "Logging Message Loop.vi"("System Control"=w4, "Data Queue"=w6, "Logging"=w31) -> ("error out"=w16:errorcluster)  [unwired: 8 in]
  n221 = Unregister For Events(event registration refnum=w23) -> (error out=w18:errorcluster)  [unwired: 1 in]
  n222 = Merge Errors(w27, w19, w18, w17, w16, w15, w14) -> (w12:errorcluster)
  n223 = call <vilib>:"Simple Error Handler.vi"("error in (no error)"=w12) -> ()  [unwired: 4 in, 5 out]
  n224 = Cluster To Array(cluster=w11) -> (array=w10:refnum<queue>[])
  n225 = for {
    shift-right: [w593] -> w9
    shift-left: w12 -> [w594]
    tunnel: w10 -> [w595] mode=indexing
    n226 = Release Queue(queue=w595, force destroy? (F)=TRUE, error in (no error)=w594) -> (error out=w593:errorcluster)  [unwired: 2 out]
  }
  n227 = call "Destroy User Event - Stop.vi"("error in (no error)"=w9, "User Event - Stop"=w22) -> ("error out"=w24:errorcluster)  [unwired: 9 in]
  n228 = disable-structure shown="RUN_TIME_ENGINE==True" {
    disable-tunnel: w24 -> [_ _]
    frame condition #0 (active) {
    }
    frame condition #1 {
      # "Call Quit LabVIEW if running as a built application."
      n229 = Quit LabVIEW() -> ()  [unwired: 1 in]
    }
  }
